vi "tunnel M2-M2.5.vi"(8 "error in (no error)":errorcluster) -> (0 "error out":errorcluster)   [LabVIEW 2017]
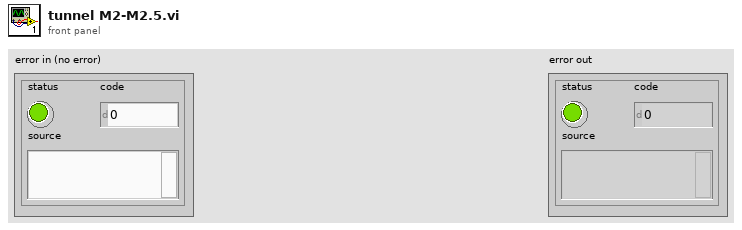
[diagram p1: front panel]
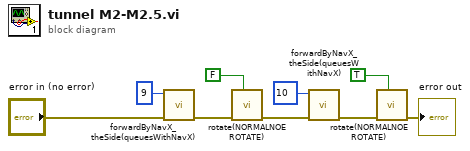
[diagram p0: block diagram]
diagram:
  n1 = call "forwardByNavX_theSide(queuesWithNavX).vi"("error in (no error)"="error in (no error)", "distance the side"=u32 9) -> ("error out"=w7:errorcluster)  [unwired: 9 in]
  n2 = call "rotate(NORMALNOE ROTATE).vi"("On/Off\nRight/Left"=FALSE ("On/Off\nRight/Left"), "error in (no error)"=w7) -> ("error out"=w6:errorcluster)  [unwired: 9 in]
  n3 = call "forwardByNavX_theSide(queuesWithNavX).vi"("error in (no error)"=w6, "distance the side"=u32 10) -> ("error out"=w5:errorcluster)  [unwired: 9 in]
  n4 = call "rotate(NORMALNOE ROTATE).vi"("On/Off\nRight/Left"=TRUE ("On/Off\nRight/Left"), "error in (no error)"=w5) -> ("error out"=→"error out":errorcluster)  [unwired: 9 in]
